vi "TestHIL.vi"() -> ()   [LabVIEW 2010]
uses:
  <vilib>/picture/picture.llb/Draw True-Color Pixmap.vi
panel:
  out "Packet Sent":string
  out "Bytes written":i32
  out "Packet Payload":string
  out "bytes read":i32
  out "Counter Send/receive":dynamicdata(graph)
  in  "Receiver port number":i32=9002
  in  "Sender port number":i32=9002
  out "KTH  Automatic Control \nTemplates. Test Bi-directional communication \nSerialForwarder-Mote":picture
  # "READ PACKET"
  # "WRITE PACKET"
  # "Communication control"
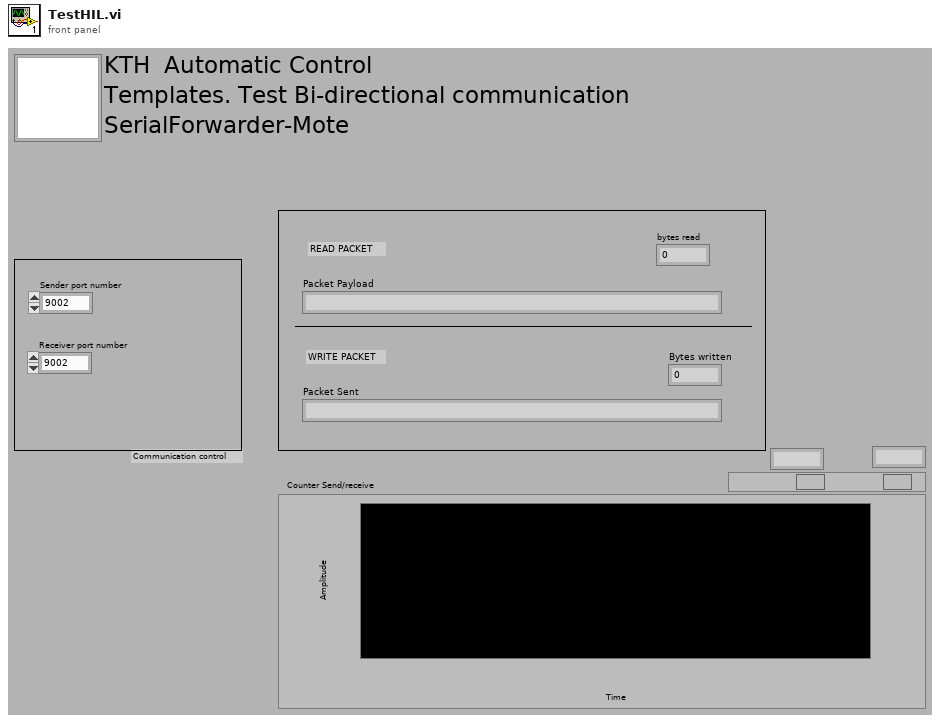
[diagram p1: front panel]
types:
  T1 = typedef "imagedata.ctl" = cluster{"image type":i32, "image depth":i32, "image":u8[], "mask":u8[], "colors":u32[], "Rectangle":cluster{"left":i16, "top":i16, "right":i16, "bottom":i16}}
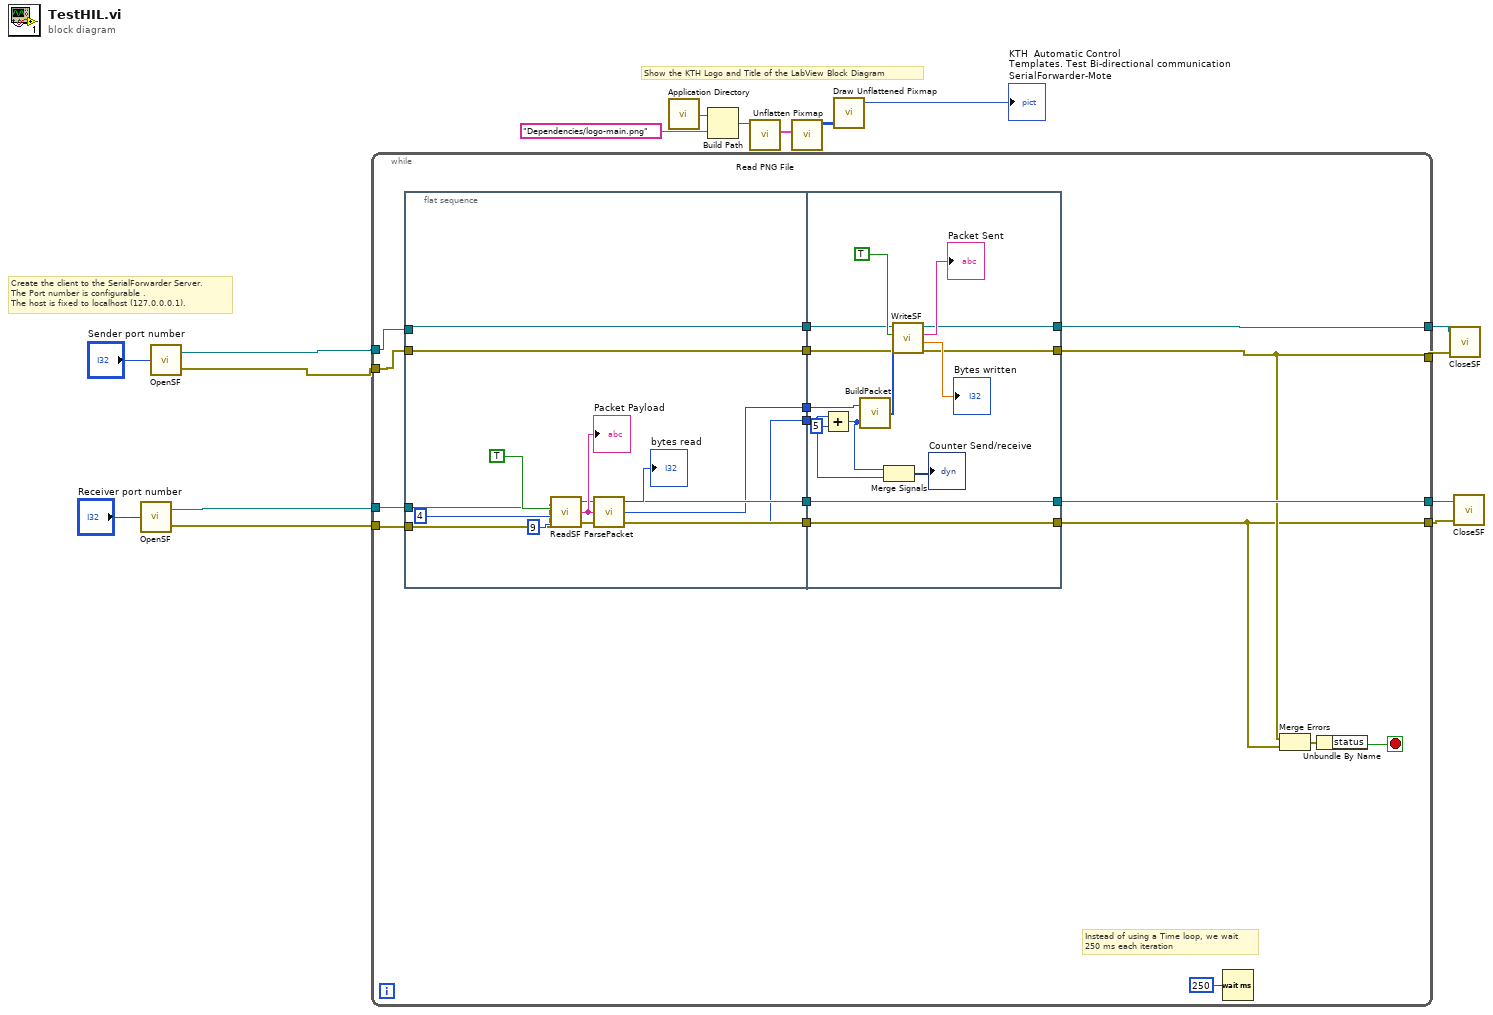
[diagram p0: block diagram]
diagram:
  # "Create the client to the SerialForwarder Server.\nThe Port number is configurable . \nThe host is fixed to localhost (127.0.0.0.1)."
  # "Show the KTH Logo and Title of the LabView Block Diagram"
  n1 = call "OpenSF.vi"("Port Number"="Receiver port number") -> ("error out"=w7:errorcluster, "connection ID"=w8:refnum<k5>)
  n2 = call "OpenSF.vi"("Port Number"="Sender port number") -> ("error out"=w1:errorcluster, "connection ID"=w2:refnum<k5>)
  n3 = while {
    tunnel: w2 -> [w18]
    tunnel: w1 -> [w17]
    tunnel: w8 -> [w27]
    tunnel: w7 -> [w26]
    tunnel: [w29] -> w6
    tunnel: [w22] -> w5
    tunnel: [w25] -> w4
    tunnel: [w21] -> w3
    stop <- w33 stop-if-true
    # "Instead of using a Time loop, we wait \n250 ms each iteration"
    n4 = flat-sequence {
      tunnel: w18 -> [w41]
      tunnel: [w41] -> w30
      tunnel: w17 -> [w40]
      tunnel: [w40] -> w28
      tunnel: w27 -> [w39]
      tunnel: w26 -> [w38]
      tunnel: [w37] -> w24
      tunnel: [w36] -> w23
      tunnel: [w35] -> w20
      tunnel: [w34] -> w19
      tunnel: w30 -> [w57]
      tunnel: [w56] -> w29
      tunnel: [w55] -> w22
      tunnel: w28 -> [w54]
      tunnel: [w53] -> w25
      tunnel: w24 -> [w53]
      tunnel: [w52] -> w21
      tunnel: w23 -> [w52]
      tunnel: w20 -> [w51]
      tunnel: w19 -> [w49]
      frame #0 {
        n5 = call "ReadSF.vi"("connection ID in"=w39, "error in"=w38, "enabled"=TRUE ("Enable Read"), "bytes to read"=4, "header size"=9 ("bytes to read")) -> ("connection ID out"=w37:refnum<k5>, "string"=w45:string, "error out"=w36:errorcluster)  [unwired: 1 in]
        "Packet Payload" <- w45
        n6 = call "ParsePacket.vi"("data out"=w45) -> ("Counter"=w34:i16, "Dummy"=w35:i16, "Bytes read"=→"bytes read":i32)
      }
      frame #1 {
        n7 = Add(x=w49, y=i16 5) -> (x+y=w48:i16)
        n8 = call "BuildPacket.vi"("Counter"=w48, "Dummy"=w51) -> ("PacketArray"=w58:i32[])
        n9 = Merge Signals(w48, w49) -> (→"Counter Send/receive":dynamicdata)
        n10 = call "WriteSF.vi"("error in"=w54, "packet"=w58, "Enablle write"=TRUE ("Enable Write"), "connection ID"=w57) -> ("error out"=w55:errorcluster, "Bytes written to SF"=→"Bytes written":dbl, "Packet String"=→"Packet Sent":string, "connection ID out"=w56:refnum<k5>)
      }
    }
    n11 = Wait (ms)(milliseconds to wait=u32 250) -> ()  [unwired: 1 out]
    n12 = Merge Errors(w22, w21) -> (w31:errorcluster)
    n13 = Unbundle By Name(w31) -> ("status"=w33:bool)
  }
  n14 = call <vilib>:"Application Directory.vi"() -> ("Application Directory"=w12:path)
  n15 = Build Path(base path=w12, name or relative path="Dependencies/logo-main.png") -> (appended path=w13:path)
  n16 = call <vilib>:"Read PNG File.vi"("path to PNG file"=w13) -> ("image data"=w16:T1)  [unwired: 8 in, 2 out]
  n17 = call <vilib>:"Unflatten Pixmap.vi"("image data"=w16) -> ("24-bit pixmap"=w15:u32[][])  [unwired: 4 in, 6 out]
  n18 = call-poly <vilib>:"Draw Unflattened Pixmap.vi"("data (RGB format)"=w15) -> ("new picture"=→"KTH  Automatic Control \nTemplates. Test Bi-directional communication \nSerialForwarder-Mote":picture)  [unwired: 8 in]
  n19 = call "CloseSF.vi"("error out"=w5, "connection ID"=w6) -> ()  [unwired: 1 in]
  n20 = call "CloseSF.vi"("error out"=w3, "connection ID"=w4) -> ()  [unwired: 1 in]
